vi "Drivebase Immediate.vi"(9 "Left Setpoint":dbl, 10 "Right Setpoint":dbl format="%#_13g") -> ()   [LabVIEW 2019]
uses:
  <vilib>/picture/picture.llb/imagedata.ctl
  Bordeaux/bordeaux-pathinator/Bordeaux/Command Stuff/Single Cmd Info.ctl
  Implementation/Drivebase Operations.ctl
  Implementation/Drivebase Setpoints.ctl
  <vilib>/Rock Robotics/WPI/Framework/Completion Status.ctl
  <vilib>/Rock Robotics/WPI/Framework/Completion Notifier.ctl
  <vilib>/Rock Robotics/WPI/Framework/Command Status Info.ctl
panel:
  in  "Description":string
  out "Command Info Out":T1
  in  "Command Info In":T1
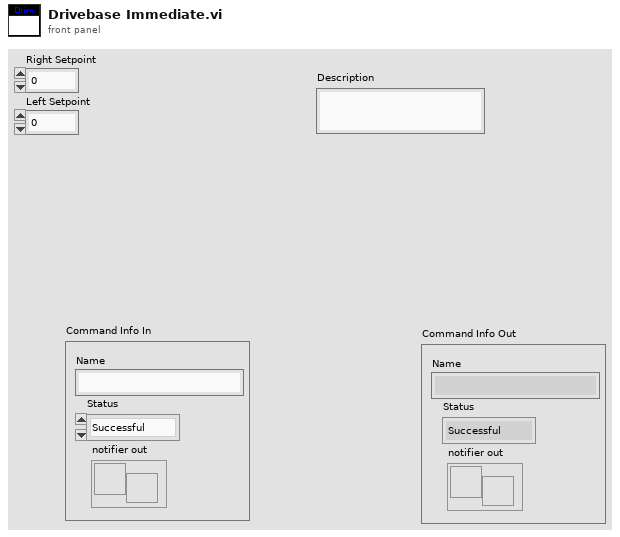
[diagram p1: front panel]
types:
  T1 = typedef "Command Status Info.ctl" = cluster{"Name":string, "Status":T2, "notifier out":T3}
  T2 = typedef "Completion Status.ctl" = enum16{"Successful", "Aborted", "Incomplete"}
  T3 = typedef "Completion Notifier.ctl" = refnum<notifier>
  T4 = typedef "Drivebase Setpoints.ctl" = cluster{"Operation":T5, "Left Setpoint":dbl, "Right Setpoint":dbl, "Velocity":dbl[], "Angles":dbl[], "Reset Gyro":bool, "Booleans":cluster{"Robot Backwards":bool, "Path Backwards":bool}, "Commands":cluster{"Time (s)":dbl, T6, bool}[]}
  T5 = typedef "Drivebase Operations.ctl" = enum16{"Reserve", "Read Current", "Immediate", "Pathinator"}
  T6 = typedef "Single Cmd Info.ctl" = cluster{"Name":string, "CPTM.DataType":variant, "All Control Values Variant":cluster{"Name":string, "Variant Data":variant}[], "icon full":T7, "icon scaled":T7, "Path":path, "Subsystem Color":u32}
  T7 = typedef "imagedata.ctl" = cluster{"image type":i32, "image depth":i32, "image":u8[], "mask":u8[], "colors":u32[], "Rectangle":cluster{"left":i16, "top":i16, "right":i16, "bottom":i16}}
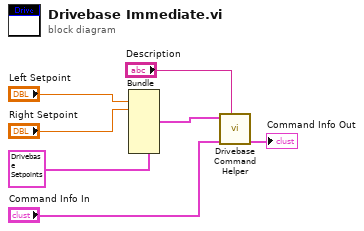
[diagram p0: block diagram]
diagram:
  n1 = Bundle(cluster=T4 {"Operation"=enum."Immediate", "Left Setpoint"=0.0, "Right Setpoint"=0.0, "Velocity"=[], "Angles"=[], "Reset Gyro"=FALSE, "Booleans"={"Robot Backwards"=FALSE, "Path Backwards"=FALSE}, "Commands"=[]} ("SubSystem Data"), "Left Setpoint"="Left Setpoint", "Right Setpoint"="Right Setpoint") -> (w3:T4)  [unwired: 6 in]
  n2 = call "Drivebase Command Helper.vi"("Description"="Description", "Command Info In"="Command Info In", "SubSystem Data"=w3) -> ("Command Info Out"=→"Command Info Out":T1)  [unwired: 6 in, 2 out]
